vi "encode_data.vi"(2 "error in":errorcluster, 3 "header size":i8=10, 4 "Cluster":cluster{"type":string, "content":string}={"type"="hello", "content"="hello again"}) -> (0 "error out":errorcluster, 1 "encode_string":string)   [LabVIEW 2018]
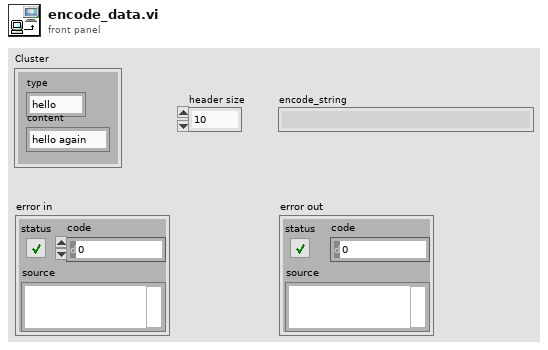
[diagram p1: front panel]
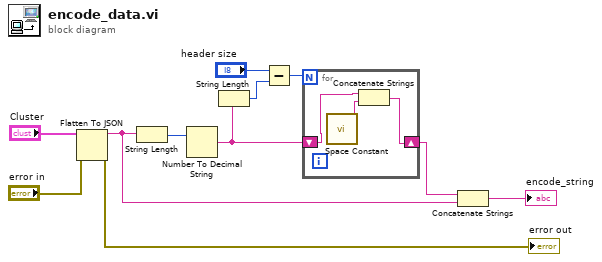
[diagram p0: block diagram]
diagram:
  n1 = Flatten To JSON(anything="Cluster", error in (no error)="error in") -> (JSON string=w3:string, 11:→"error out":errorcluster)  [unwired: 1 in]
  n2 = String Length(string=w3) -> (length=w7:i32)
  n3 = Number To Decimal String(number=w7) -> (decimal integer string=w6:string)  [unwired: 1 in]
  n4 = String Length(string=w6) -> (length=w5:i32)
  n5 = Subtract(x="header size", y=w5) -> (x-y=w8:i32)
  n6 = for {
    N: w8 -> [_]
    shift-right: [w14] -> w4
    shift-left: w6 -> [w13]
    n7 = call <vilib>:"Space Constant.vi"() -> ("String"=w12:string)
    n8 = Concatenate Strings(w13, w12) -> (w14:string)
  }
  n9 = Concatenate Strings(w4, w3) -> (→"encode_string":string)
